vi "sc5511a_soft_front_panel.vi"() -> ()   [LabVIEW 2010]
panel:
  out "message":string="List/Sweep Mode Disabled"
  out "Selected Resource":string
  out "On":bool
  in  "stop":bool
  in  "Tab Control":T1(tab)
  in  "Spur Suppression":u8(ring) items=["Enabled", "Disabled"]
  in  "AutoLevel":u8(ring) items=["Enable", "Disable"]
  in  "Loop Gain":u8(ring) items=["Normal", "Low"]
  in  "Ref. Out Freq":u8(ring) items=["10 MHz", "100 MHz"]
  in  "Ref. Clock Source":u8(ring) items=["Internal 10 MHz", "Lock to External"]
  in  "RF1 Standby":bool
  in  "Lock Mode":u8(ring) items=["Harmonic Lock", "Frac-N Lock"]
  in  "ALC MODE":u8(ring) items=["Closed", "Opened"]
  in  "Power":sgl=30.0 min=-40 max=30 format="%.2f"
  in  "Interval (s)":u16=5
  in  "GetStatus":bool
  in  "Trigger":bool
  out "Device Status":T2={"Synth Mode"=1, "RF Out"=0, "Auto Level"=0, "ALC Mode"=1, "Standby"=1, "Rf RF Mode"=0, "List Mode State"=0, "RF2 Standby"=0, "Ref Lock Enable"=1, "Ext Ref Detected"=1, "Ref out mode"=1, "Main PLL"=1, "Crs PLL"=1, "Fine PLL"=1, "device accessed"=0, "Over Temp"=0, "MainLED"=FALSE, "CrsLED"=FALSE, "FineLED"=FALSE} {"Over Temp" items=["Normal", "Over Temp"]; "Ref out mode" items=["10 MHz", "100 MHz"]; "device accessed" items=["NO", "YES"]; "RF2 Standby" items=["Disabled", "Enabled"]; "Standby" items=["Disable", "Enabled"]; "Auto Level" items=["Enable", "Disable"]; "Ext Ref Detected" items=["Not Detected", "Detected"]; "Ref Lock Enable" items=["Disabled", "Enabled"]; "RF Out" items=["Disabled", "Enabled"]; "ALC Mode" items=["Closed", "Opened"]; "Rf RF Mode" items=["Single Tone", "List/Sweep"]; "Synth Mode" items=["Harmonic", "FracN"]; "List Mode State" items=["Not Triggered", "Triggered"]; "Main PLL" items=["NOT Locked", "Locked"]; "Crs PLL" items=["NOT Locked", "Locked"]; "Fine PLL" items=["NOT Locked", "Locked"]}
  in  "RF Frequency":dbl=2005000000.0 min=80000000.0 max=21000000000.0 step=1.0 format="%.9p"
  in  "RF Mode":u8(ring) items=["Single Tone", "List/Sweep"]
  in  "RF Enable":bool
  in  "RF2 Freq":sgl=6000.0 min=25 max=6000 step=25
  in  "RF2 Standby":bool
  in  "Set As Default":bool
  in  "Dwell Period (ms)":dbl=10.0 min=0.0 step=0.5 format="%.1f"
  in  "Sweep/List Cycles":u32
  in  "Sweep Freq Parameter":T3={"Start Frequency"=10040000000, "Stop Frequency"=10050000000, "Step Frequency"=100000} {"Step Frequency" max=6500000000 format="%.9p"; "Stop Frequency" max=21000000000 format="%.9p"; "Start Frequency" format="%.9p"}
  in  "List Mode Config":T4={"Sweep / List"=1, "Direction"=0, "Shape"=1, "Trigger Source"=1, "HW Trigger Mode"=0, "Return to Start"=0, "Trigger Out State"=1, "Trigger Out Behavior"=0} {"Trigger Out Behavior" items=["Trigger On Step", "Trigger On Cycle"]; "Trigger Out State" items=["Trigger Out Disable", "Trigger Out Enable"]; "Return to Start" items=["Stop at End", "Return to Start"]; "HW Trigger Mode" items=["Start/Stop", "Step"]; "Trigger Source" items=["Software", "Hardware"]; "Shape" items=["Sawtooth", "Triangle"]; "Direction" items=["Low to High", "High to Low"]; "Sweep / List" items=["List", "Sweep (start/stop/step)"]}
  in  "Load Config":bool
  in  "Save Buffer to EEPROM":bool
  in  "Read EEPROM to Buffer":bool
  in  "Download to Buffer":bool
  in  "Read From File":bool
  in  "Frequency List (2048 max)":u64[](array[numeric]) format="%.9p"
  out "message 2":string
  out "List Points":u32
  in  "SelfCal":bool
  out "Temperature":sgl=40.0 min=-30 max=120 format="%.1f"
  out "Device Info":T5={"Product SN"=268435879, "Hardware Rev"=2.0, "Firmware Rev"=2.0, "Manuf Date"={"Year"=14, "Month"=9, "Day"=10, "Hour"=10}} {"Firmware Rev" format="%.2g"; "Hardware Rev" format="%.2g"; "Product SN" format="%.0x"}
  out "error out":errorcluster
  # "MHz"
  # "Program will stop and the device will \nreinitialize after self calibration"
  # "DegC"
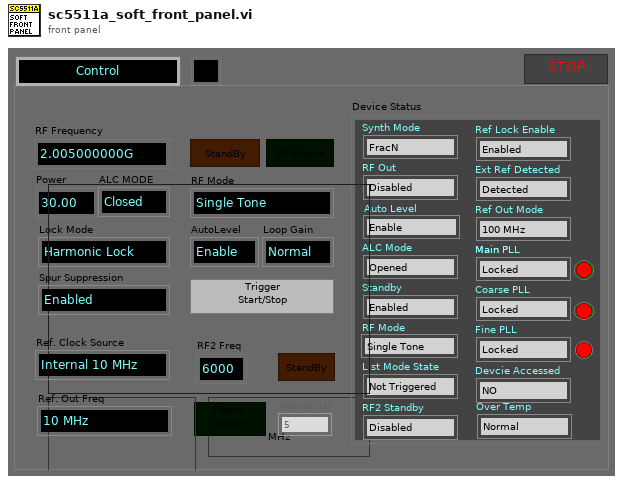
[diagram p1: front panel]
types:
  T1 = enum32{"Control", "Config Sweep/List", "List Entry", "Device Info"}
  T2 = cluster{"Synth Mode":u16, "RF Out":u16, "Auto Level":u16, "ALC Mode":u16, "Standby":u16, "Rf RF Mode":u16, "List Mode State":u16, "RF2 Standby":u16, "Ref Lock Enable":u16, "Ext Ref Detected":u16, "Ref out mode":u16, "Main PLL":u8, "Crs PLL":u8, "Fine PLL":u8, "device accessed":u16, "Over Temp":u16, "MainLED":bool, "CrsLED":bool, "FineLED":bool}
  T3 = cluster{"Start Frequency":u64, "Stop Frequency":u64, "Step Frequency":u64}
  T4 = cluster{"Sweep / List":u8, "Direction":u8, "Shape":u8, "Trigger Source":u8, "HW Trigger Mode":u8, "Return to Start":u8, "Trigger Out State":u8, "Trigger Out Behavior":u8}
  T5 = cluster{"Product SN":u32, "Hardware Rev":sgl, "Firmware Rev":sgl, "Manuf Date":cluster{"Year":u8, "Month":u8, "Day":u8, "Hour":u8}}
  T6 = cluster{"Product SN":u32, "Hardware Rev":sgl, "Firmware Rev":sgl, "Manuf Date":cluster{"Year":u32, "Month":u32, "Day":u32, "hour":u32}}
  T7 = enum32{"Control", "Config Sweep/List", "List Entry"}
  T8 = enum8{"Enabled", "Disabled", "Disabled and Grayed Out"}
  T9 = cluster{"Synth Mode":u16, "RF Out":u16, "Auto Power":u16, "ALC Mode":u16, "Standby":u16, "Rf RF Mode":u16, "List Mode State":u16, "RF2 Standby":u16, "Ref Lock Enable":u16, "Ext Ref Detected":u16, "Ref out mode":u16, "Main PLL":u8, "Crs PLL":u8, "Fine PLL":u8, "device accessed":u16, "Over Temp":u16, "MainLED":bool, "CrsLED":bool, "FineLED":bool}
  T10 = cluster{"Product SN":u32, "Hardware Rev":sgl, "Firmware Rev":sgl, "Manufacture Date":cluster{"Year":u8, "Month":u8, "Day":u8, "hour":u8}}
  T11 = cluster{"List Mode Config":cluster{"List/SSS":u8, "Direction":u8, "Shape":u8, "Trigger Source":u8, "HW Trigger Mode":u8, "Return to Start":u8, "Trigger Out State":u8, "Trigger Out Behavior":u8}, "Operate Status":cluster{"Lock Mode":u8, "Loop Gain":u8, "Device Accessed":u8, "RF2 Standby":u8, "RF1 Standby":u8, "AutoPwrLevel":u8, "AlcMode":u8, "RFOutState":u8, "Ref Lock Enable":u8, "ExtRefDetected":u8, "RefOutSelect":u8, "ListRuning":u8, "RF Mode":u8, "OverTempStatus":u8, "Harmonic_SS":u8}, "PLL Status":cluster{"Sum PLL":u8, "Crs PLL":u8, "Fine PLL":u8, "Crs Ref PLL":u8, "Crs assist PLL":u8, "Ref Clk PLL":u8, "Clk 10 PLL":u8, "Lo2 PLL":u8}}
  T12 = cluster{"RF1 Freq":u64, "Sweep Start Freq":u64, "Sweep Stop Freq":u64, "Sweep Step Freq":u64, "Sweep dwell time (.5ms)":u32, "Sweep Cycles":u32, "List Buffer Points":u32, "RF1 Level (dBm)":sgl, "RF2 freq":u16}
  T13 = cluster{"List/SSS":u8, "Direction":u8, "Shape":u8, "Trigger Source":u8, "HW Trigger Mode":u8, "Return to Start":u8, "Trigger Out State":u8, "Trigger Out Behavior":u8}
  T14 = cluster{"Sweep Start Freq":u64, "Sweep Stop Freq":u64, "Sweep Step Freq":u64}
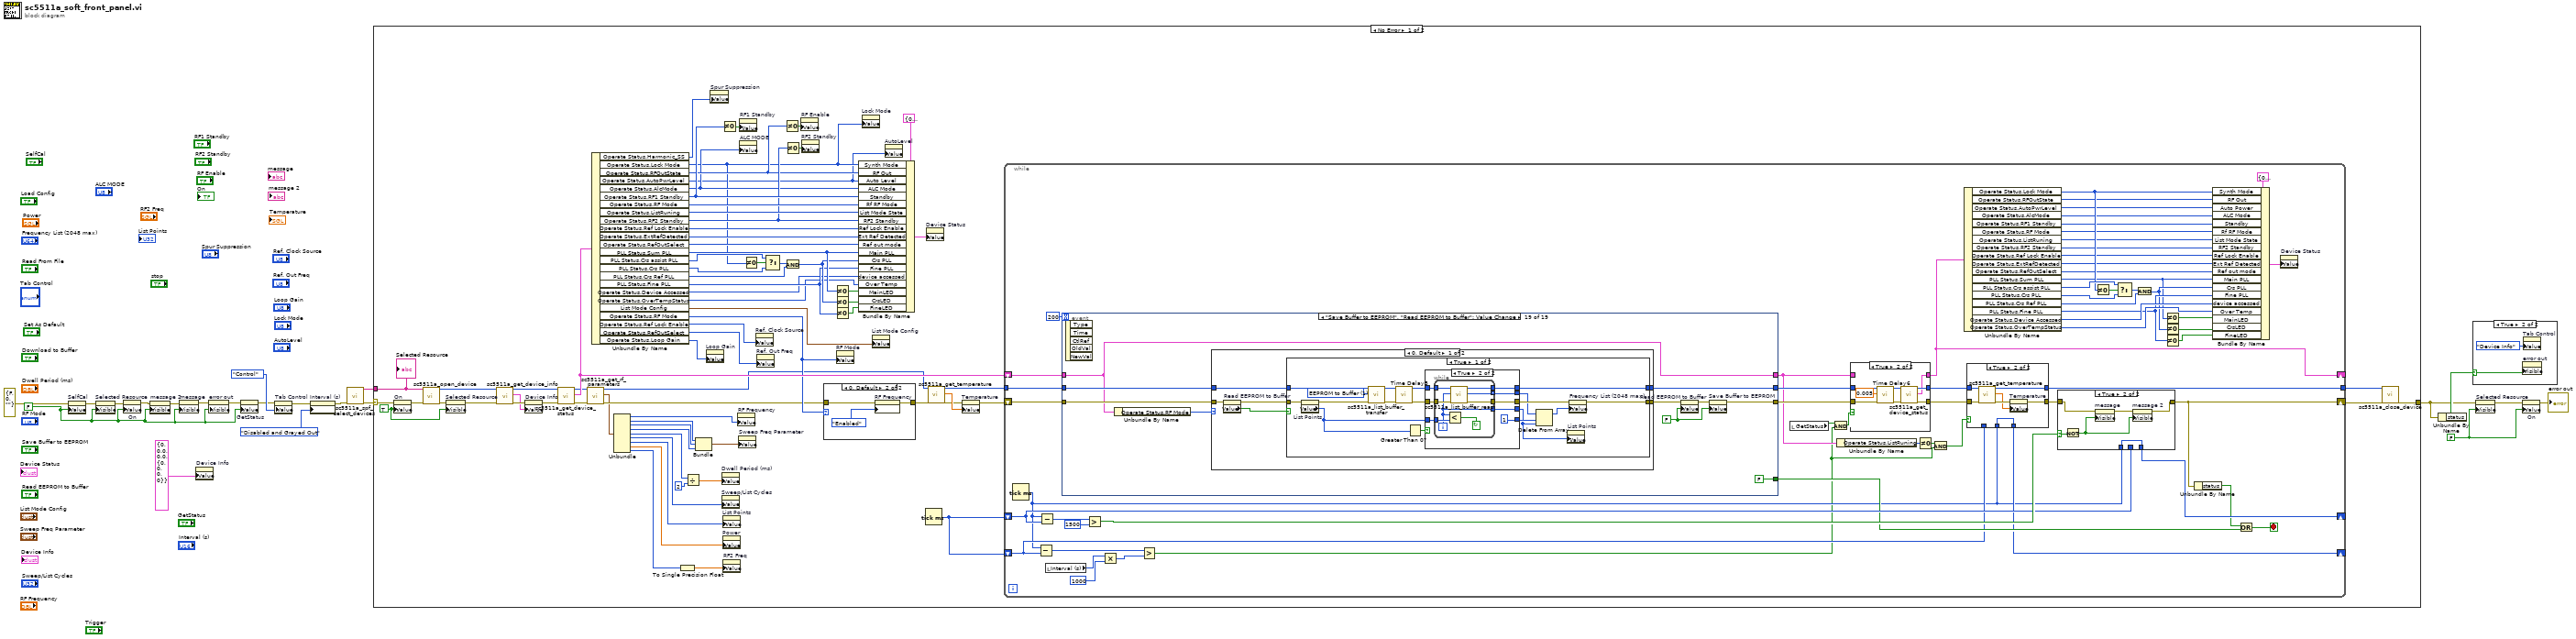
[diagram p0: block diagram]
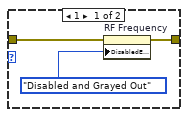
[diagram p3: hidden frame]
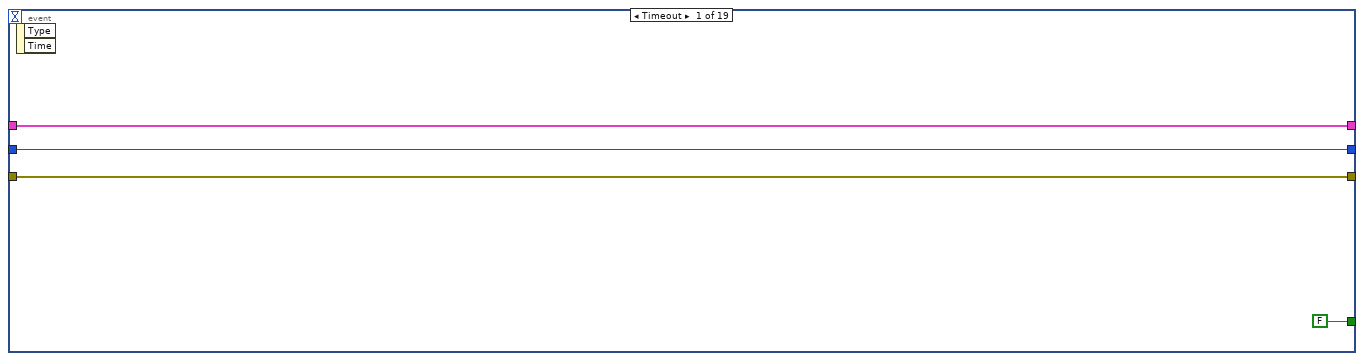
[diagram p7: hidden frame]
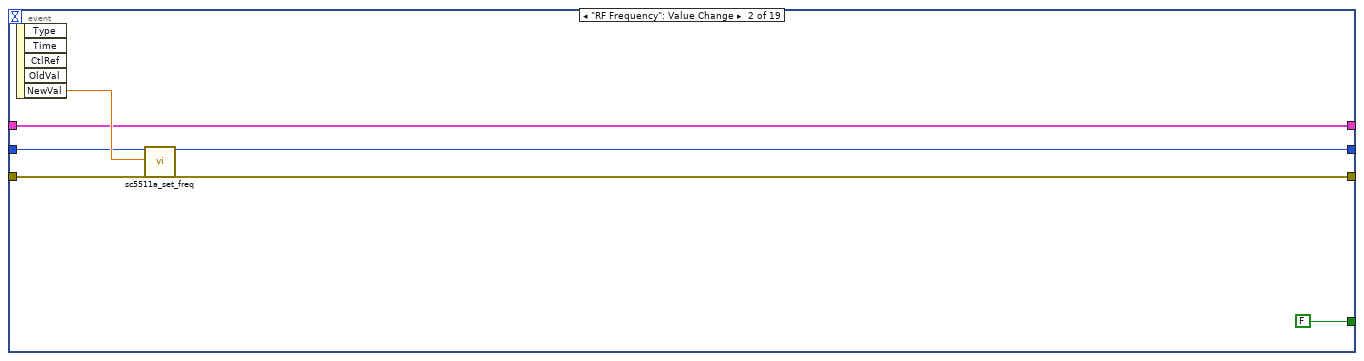
[diagram p8: hidden frame]
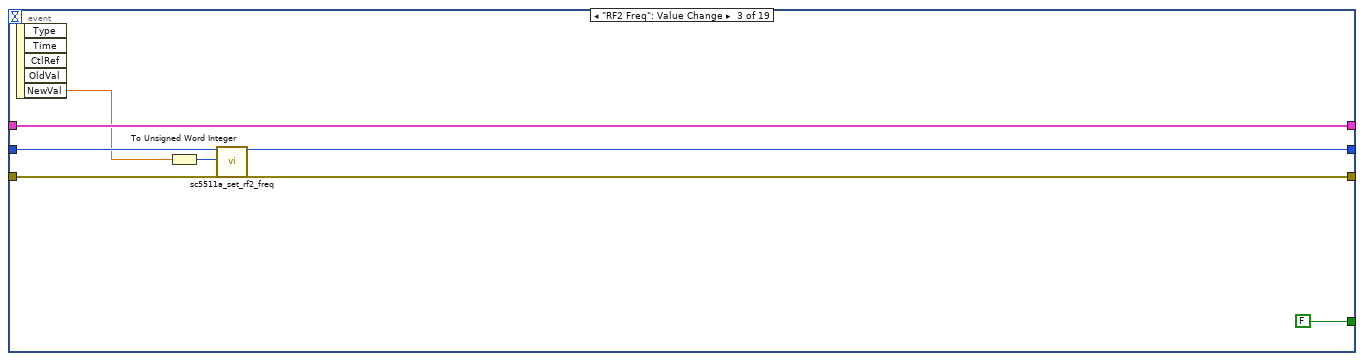
[diagram p9: hidden frame]
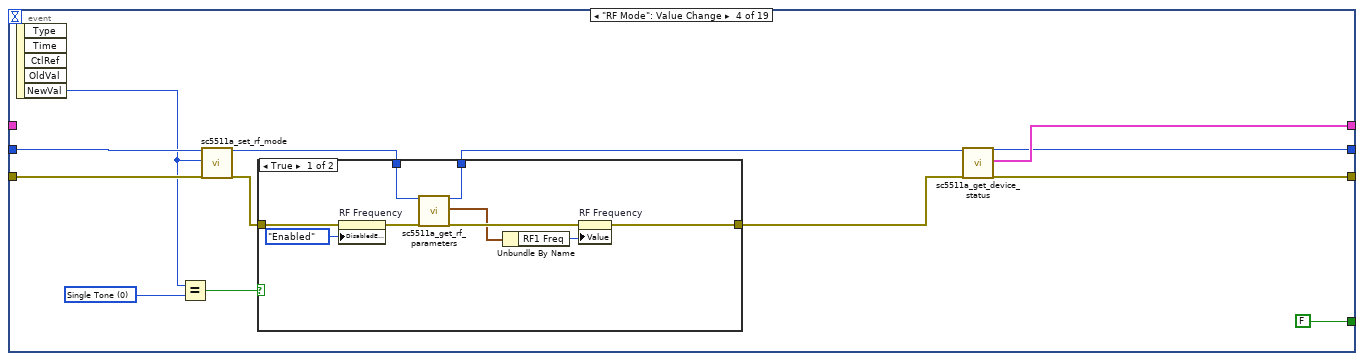
[diagram p10: hidden frame]
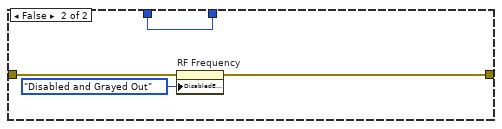
[diagram p11: hidden frame]
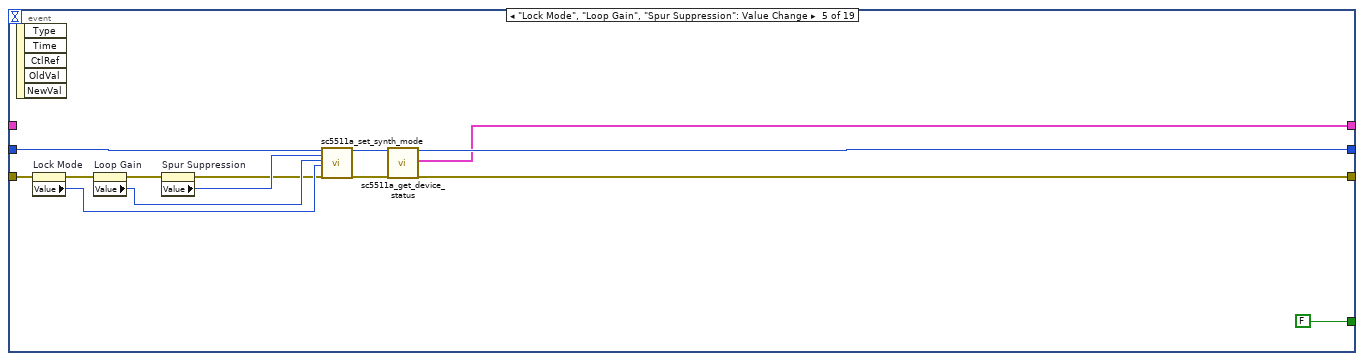
[diagram p12: hidden frame]
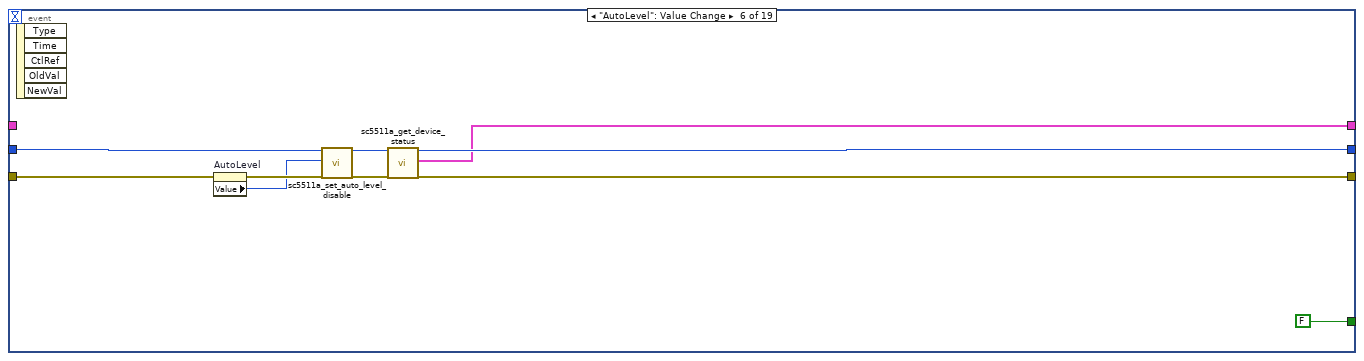
[diagram p13: hidden frame]
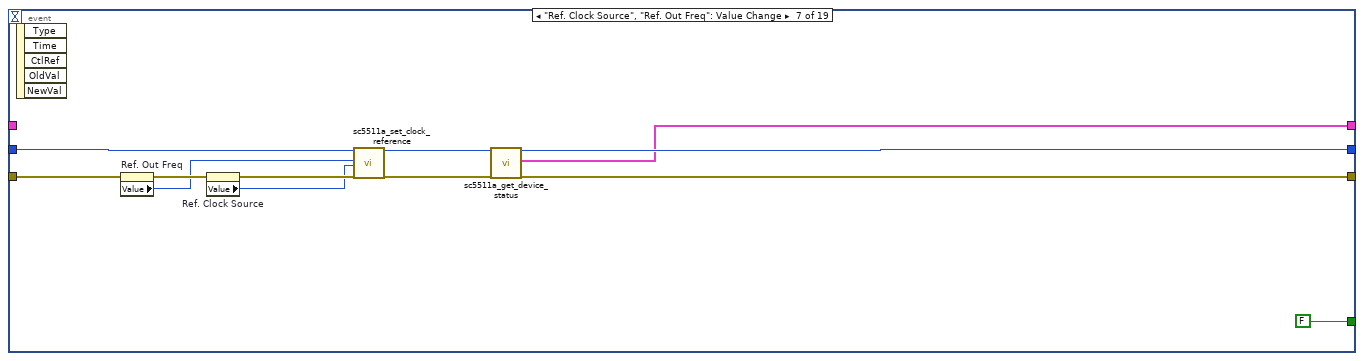
[diagram p14: hidden frame]
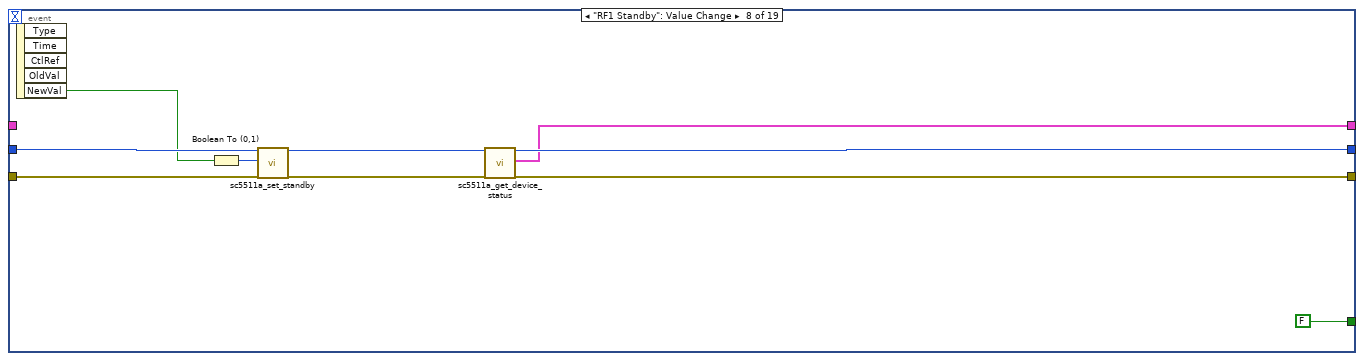
[diagram p15: hidden frame]
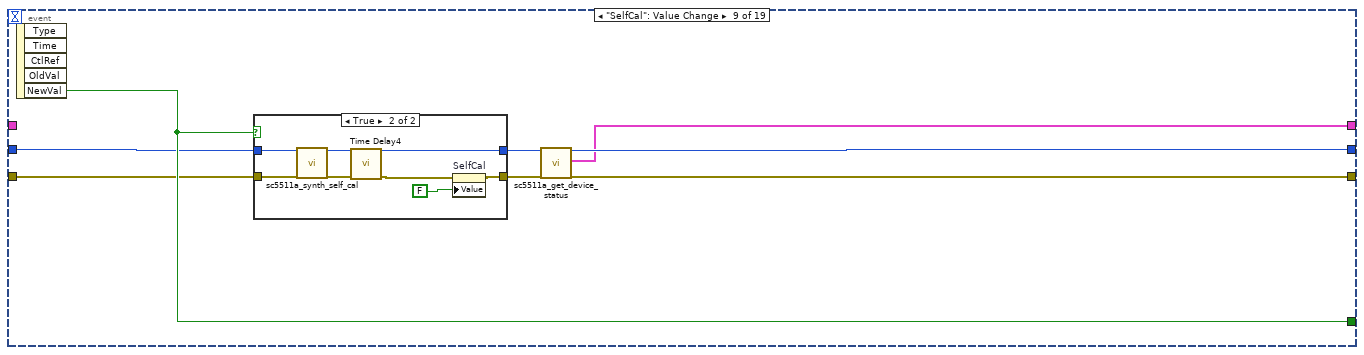
[diagram p16: hidden frame]
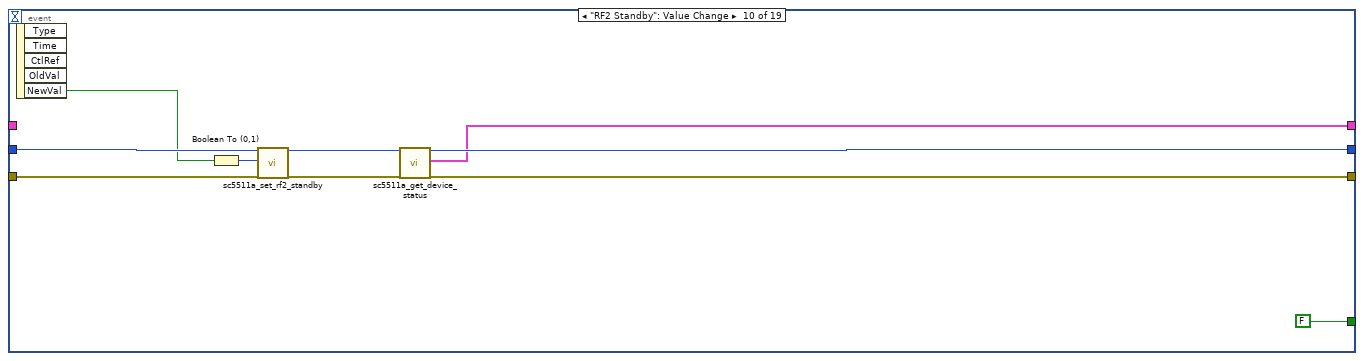
[diagram p18: hidden frame]
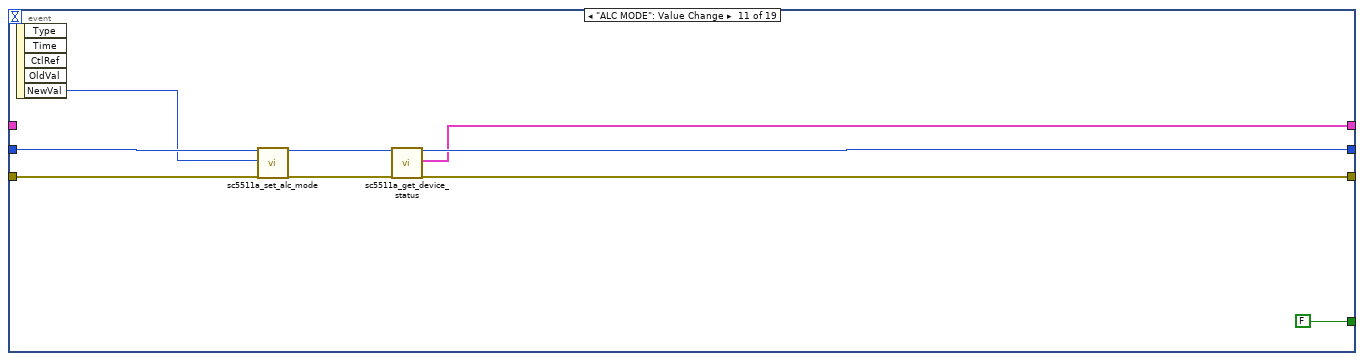
[diagram p19: hidden frame]
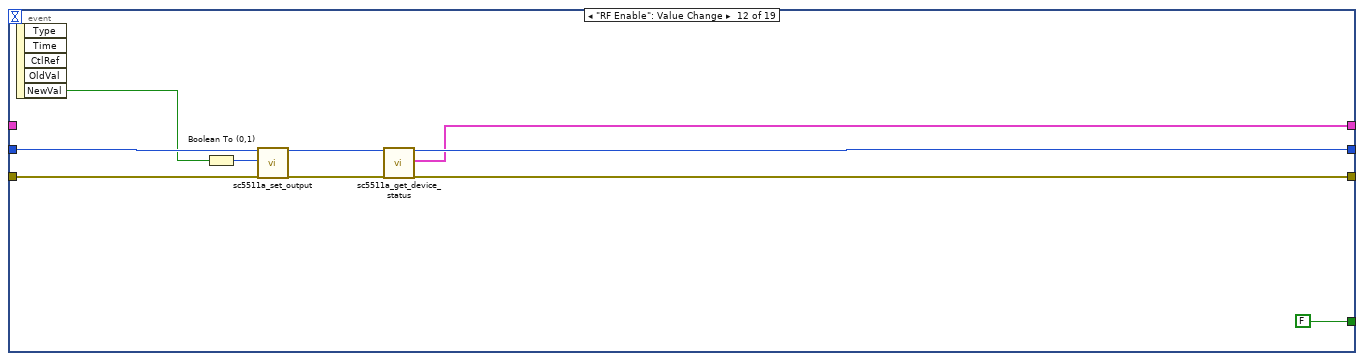
[diagram p20: hidden frame]
diagram:
  w4 = FALSE ("Visible")
  w2 = FALSE ("Visible")
  n1 = property on="SelfCal" class="Bool (strict)"(error in=errorcluster {"status"=FALSE, "code"=0, "source"=""} ("error in (no error)"), "Value"=w2) -> (error out=w3:errorcluster)  [unwired: 1 in, 1 out]
  n2 = property on="Selected Resource" class="Str"(error in=w3, "Visible"=w2) -> (error out=w7:errorcluster)  [unwired: 1 in, 1 out]
  n3 = property on="On" class="Bool (strict)"(error in=w7, "Value"=w2) -> (error out=w12:errorcluster)  [unwired: 1 in, 1 out]
  n4 = property on="message 2" class="Str"(error in=w12, "Visible"=w2) -> (error out=w21:errorcluster)  [unwired: 1 in, 1 out]
  n5 = property on="message" class="Str"(error in=w21, "Visible"=w2) -> (error out=w20:errorcluster)  [unwired: 1 in, 1 out]
  n6 = property on="Device Info" class="Clust (strict)"("Value"=T6 {"Product SN"=0, "Hardware Rev"=0.0, "Firmware Rev"=0.0, "Manuf Date"={"Year"=0, "Month"=0, "Day"=0, "hour"=0}} ("Device Info")) -> ()  [unwired: 2 in, 2 out]
  n7 = property on="error out" class="Clust (strict)"(error in=w20, "Visible"=w2) -> (error out=w19:errorcluster)  [unwired: 1 in, 1 out]
  n8 = property on="GetStatus" class="Bool (strict)"(error in=w19, "Value"=w2) -> (error out=w15:errorcluster)  [unwired: 1 in, 1 out]
  n9 = property on="Tab Control" class="TabCtl (strict)"(error in=w15, "Value"=T7."Control" ("Tab Control")) -> (error out=w16:errorcluster)  [unwired: 1 in, 1 out]
  n10 = property on="Interval (s)" class="DigNum (strict)"(error in=w16, "DisabledEnum"=T8."Disabled and Grayed Out" ("Disabled")) -> (error out=w9:errorcluster)  [unwired: 1 in, 1 out]
  n11 = call "sc5511a_spf_select_devices.vi"("error in (no error)"=w9) -> ("Selected Resource"=w8:string, "error out"=w10:errorcluster)  [unwired: 17 in]
  n12 = case shown="No Error" w10 {
    selector: w10 -> [w80 w556]
    tunnel: [w93 w556] -> w6
    tunnel: w8 -> [w79 _]
    frame No Error {
      w23 = TRUE ("Visible")
      n13 = property on="On" class="Bool (strict)"(error in=w80, "Value"=w23) -> (error out=w81:errorcluster)  [unwired: 1 in, 1 out]
      n14 = call "sc5511a_open_device.vi"("COM (String) eg COM1"=w79, "error in (no error)"=w81) -> ("deviceHandle"=w83:u32, "error out"=w25:errorcluster)  [unwired: 16 in]
      n15 = property on="Selected Resource" class="Str"(error in=w25, "Visible"=w23) -> (error out=w24:errorcluster)  [unwired: 1 in, 1 out]
      n16 = call "sc5511a_get_device_info.vi"("deviceHandle"=w83, "error in"=w24) -> ("deviceHandle"=w90:u32, "Device Info"=w75:T10, "error out"=w89:errorcluster)  [unwired: 15 in]
      n17 = property on="Device Info" class="Clust (strict)"(error in=w89, "Value"=w75) -> (error out=w88:errorcluster)  [unwired: 1 in, 1 out]
      n18 = call "sc5511a_get_device_status.vi"("deviceHandle"=w90, "error in"=w88) -> ("deviceHandle"=w76:u32, "Device Status"=w91:T11, "error out"=w78:errorcluster)  [unwired: 15 in]
      n19 = call "sc5511a_get_rf_parameters.vi"("deviceHandle"=w76, "error in"=w78) -> ("deviceHandle"=w36:u32, "RF Params"=w74:T12, "error out"=w77:errorcluster)  [unwired: 15 in]
      n20 = Unbundle By Name(w91) -> ("Operate Status.Harmonic_SS"=w22:u8, "Operate Status.Lock Mode"=w29:u8, "Operate Status.RFOutState"=w38:u8, "Operate Status.AutoPwrLevel"=w26:u8, "Operate Status.AlcMode"=w37:u8, "Operate Status.RF1 Standby"=w43:u8, "Operate Status.RF Mode"=w60:u8, "Operate Status.ListRuning"=w59:u8, "Operate Status.RF2 Standby"=w39:u8, "Operate Status.Ref Lock Enable"=w58:u8, "Operate Status.ExtRefDetected"=w57:u8, "Operate Status.RefOutSelect"=w56:u8, "PLL Status.Sum PLL"=w55:u8, "PLL Status.Crs assist PLL"=w51:u8, "PLL Status.Crs PLL"=w50:u8, "PLL Status.Crs Ref PLL"=w52:u8, "PLL Status.Fine PLL"=w48:u8, "Operate Status.Device Accessed"=w47:u8, "Operate Status.OverTempStatus"=w46:u8, "List Mode Config"=w92:T13, "Operate Status.RF Mode"=w82:u8, "Operate Status.Ref Lock Enable"=w45:u8, "Operate Status.RefOutSelect"=w44:u8, "Operate Status.Loop Gain"=w30:u8)
      n21 = Unbundle(w74) -> ("RF1 Freq"=w73:u64, "Sweep Start Freq"=w71:u64, "Sweep Stop Freq"=w70:u64, "Sweep Step Freq"=w69:u64, "Sweep dwell time (.5ms)"=w66:u32, "Sweep Cycles"=w68:u32, "List Buffer Points"=w64:u32, "RF1 Level (dBm)"=w63:sgl, "RF2 freq"=w61:u16)
      n22 = To Single Precision Float(number=w61) -> (single precision float=w62:sgl)
      n23 = Divide(x=w66, y=u32 2) -> (x/y=w67:dbl)
      n24 = Bundle("Sweep Start Freq"=w71, "Sweep Stop Freq"=w70, "Sweep Step Freq"=w69) -> (w72:T14)  [unwired: 1 in]
      n25 = property on="Loop Gain" class="Ring (strict)"("Value"=w30) -> ()  [unwired: 2 in, 2 out]
      n26 = property on="Spur Suppression" class="Ring (strict)"("Value"=w22) -> ()  [unwired: 2 in, 2 out]
      n27 = Not Equal To 0?(x=w43) -> (x != 0?=w42:bool)
      n28 = property on="Dwell Period (ms)" class="DigNum (strict)"("Value"=w67) -> ()  [unwired: 2 in, 2 out]
      n29 = property on="Sweep/List Cycles" class="DigNum (strict)"("Value"=w68) -> ()  [unwired: 2 in, 2 out]
      n30 = property on="Power" class="DigNum (strict)"("Value"=w63) -> ()  [unwired: 2 in, 2 out]
      n31 = property on="List Points" class="DigNum (strict)"("Value"=w64) -> ()  [unwired: 2 in, 2 out]
      n32 = property on="RF2 Freq" class="DigNum (strict)"("Value"=w62) -> ()  [unwired: 2 in, 2 out]
      n33 = property on="RF Frequency" class="DigNum (strict)"("Value"=w73) -> ()  [unwired: 2 in, 2 out]
      n34 = property on="Sweep Freq Parameter" class="Clust (strict)"("Value"=w72) -> ()  [unwired: 2 in, 2 out]
      n35 = property on="RF1 Standby" class="Bool (strict)"("Value"=w42) -> ()  [unwired: 2 in, 2 out]
      n36 = property on="ALC MODE" class="Ring (strict)"("Value"=w37) -> ()  [unwired: 2 in, 2 out]
      n37 = Not Equal To 0?(x=w29) -> (x != 0?=w54:bool)
      n38 = property on="Ref. Clock Source" class="Ring (strict)"("Value"=w45) -> ()  [unwired: 2 in, 2 out]
      n39 = property on="Ref. Out Freq" class="Ring (strict)"("Value"=w44) -> ()  [unwired: 2 in, 2 out]
      n40 = Select(t=w51, s=w54, f=w50) -> (s? t:f=w53:u8)
      n41 = Not Equal To 0?(x=w38) -> (x != 0?=w41:bool)
      n42 = Not Equal To 0?(x=w39) -> (x != 0?=w40:bool)
      n43 = And(x=w53, y=w52) -> (x .and. y?=w49:u8)
      n44 = property on="RF Enable" class="Bool (strict)"("Value"=w41) -> ()  [unwired: 2 in, 2 out]
      n45 = property on="RF2 Standby" class="Bool (strict)"("Value"=w40) -> ()  [unwired: 2 in, 2 out]
      n46 = case shown="0, Default" w82 {
        tunnel: w77 -> [w97 w100]
        tunnel: [w96 w99] -> w34
        frame 1 {
          n47 = property on="RF Frequency" class="DigNum (strict)"(error in=w97, "DisabledEnum"=T8."Disabled and Grayed Out" ("Disabled")) -> (error out=w96:errorcluster)  [unwired: 1 in, 1 out]
        }
        frame 0, Default {
          n48 = property on="RF Frequency" class="DigNum (strict)"(error in=w100, "DisabledEnum"=T8."Enabled" ("Disabled")) -> (error out=w99:errorcluster)  [unwired: 1 in, 1 out]
        }
      }
      n49 = Not Equal To 0?(x=w55) -> (x != 0?=w86:bool)
      n50 = Not Equal To 0?(x=w49) -> (x != 0?=w85:bool)
      n51 = Not Equal To 0?(x=w48) -> (x != 0?=w84:bool)
      n52 = property on="RF Mode" class="Ring (strict)"("Value"=w82) -> ()  [unwired: 2 in, 2 out]
      n53 = Bundle By Name(cluster=T2 {"Synth Mode"=0, "RF Out"=1, "Auto Level"=1, "ALC Mode"=0, "Standby"=0, "Rf RF Mode"=0, "List Mode State"=0, "RF2 Standby"=1, "Ref Lock Enable"=0, "Ext Ref Detected"=0, "Ref out mode"=0, "Main PLL"=1, "Crs PLL"=1, "Fine PLL"=1, "device accessed"=1, "Over Temp"=0, "MainLED"=TRUE, "CrsLED"=TRUE, "FineLED"=TRUE} ("Device Status"), "Synth Mode"=w29, "RF Out"=w38, "Auto Level"=w26, "ALC Mode"=w37, "Standby"=w43, "Rf RF Mode"=w60, "List Mode State"=w59, "RF2 Standby"=w39, "Ref Lock Enable"=w58, "Ext Ref Detected"=w57, "Ref out mode"=w56, "Main PLL"=w55, "Crs PLL"=w49, "Fine PLL"=w48, "device accessed"=w47, "Over Temp"=w46, "MainLED"=w86, "CrsLED"=w85, "FineLED"=w84) -> (w28:T2)
      n54 = property on="Lock Mode" class="Ring (strict)"("Value"=w29) -> ()  [unwired: 2 in, 2 out]
      n55 = property on="List Mode Config" class="Clust (strict)"("Value"=w92) -> ()  [unwired: 2 in, 2 out]
      n56 = property on="AutoLevel" class="Ring (strict)"("Value"=w26) -> ()  [unwired: 2 in, 2 out]
      n57 = Tick Count (ms)() -> (millisecond timer value=w87:u32)
      n58 = property on="Device Status" class="Clust (strict)"("Value"=w28) -> ()  [unwired: 2 in, 2 out]
      n59 = call "sc5511a_get_temperature.vi"("deviceHandle"=w36, "error in"=w34) -> ("deviceHandle"=w35:u32, "temperature"=w33:sgl, "error out"=w31:errorcluster)  [unwired: 15 in]
      n60 = property on="Temperature" class="DigNum (strict)"(error in=w31, "Value"=w33) -> (error out=w32:errorcluster)  [unwired: 1 in, 1 out]
      n61 = while {
        shift-right: [w143] -> w95
        shift-left: w32 -> [w161]
        tunnel: w35 -> [w160]
        tunnel: [w110] -> w94
        shift-right: [w118] -> _
        shift-left: w91 -> [w157]
        shift-right: [w147] -> _
        shift-left: w87 -> [w146]
        shift-right: [w113] -> _
        shift-left: w87 -> [w114]
        stop <- w142 stop-if-true
        n62 = Tick Count (ms)() -> (millisecond timer value=w112:u32)
        n63 = Subtract(x=w112, y=w114) -> (x-y=w151:u32)
        n64 = Subtract(x=w112, y=w146) -> (x-y=w156:u32)
        n65 = local read "Interval (s)"() -> (w152:u16)
        n66 = event shown="[18] \"Save Buffer to EEPROM\", \"Read EEPROM to Buffer\": Value Change" {
          selector: _ -> [_ _ _ _ _ _ _ _ _ _ _ _ _ _ _ _ _ _ _]
          dyn-events: _ -> [_ _ _ _ _ _ _ _ _ _ _ _ _ _ _ _ _ _ _]
          timeout: 200 -> [_ _ _ _ _ _ _ _ _ _ _ _ _ _ _ _ _ _ _]
          tunnel: w160 -> [w192 w199 w208 w219 w247 w257 w269 w278 w284 w305 w314 w324 w330 w335 w356 w367 w439 w454 w501]
          tunnel: w161 -> [w193 w198 w207 w220 w241 w249 w268 w279 w283 w306 w315 w325 w331 w340 w353 w368 w438 w455 w502]
          tunnel: [w192 w196 w205 w211 w244 w254 w260 w273 w287 w301 w310 w319 w329 w336 w356 w360 w415 w453 w496] -> w159
          tunnel: [w193 w197 w206 w212 w246 w256 w263 w274 w288 w302 w312 w321 w328 w337 w354 w362 w413 w452 w497] -> w158
          tunnel: w157 -> [w191 w195 w204 _ _ _ _ _ _ _ _ _ w333 _ w357 w363 w411 w447 w494]
          tunnel: [w191 w195 w204 w214 w242 w252 w259 w271 w286 w298 w308 w317 w333 w334 w357 w358 w411 w447 w494] -> w107
          tunnel: [FALSE ("NewVal") FALSE FALSE FALSE FALSE FALSE FALSE FALSE w285 FALSE FALSE FALSE FALSE FALSE TRUE ("NewVal") FALSE ("NewVal") FALSE ("NewVal") FALSE ("NewVal") FALSE ("NewVal")] -> w145
          event Timeout {
            n67 = event-data() -> ()  [unwired: 1 in, 2 out]
          }
          event "RF Frequency": Value Change {
            n68 = event-data() -> ("NewVal"=w200:dbl)  [unwired: 1 in, 4 out]
            n69 = call "sc5511a_set_freq.vi"("deviceHandle"=w199, "RF1 frequency"=w200, "error in"=w198) -> ("deviceHandle"=w196:u32, "error out"=w197:errorcluster)  [unwired: 15 in]
          }
          event "RF2 Freq": Value Change {
            n70 = event-data() -> ("NewVal"=w201:sgl)  [unwired: 1 in, 4 out]
            n71 = To Unsigned Word Integer(number=w201) -> (unsigned 16bit integer=w202:u16)
            n72 = call "sc5511a_set_rf2_freq.vi"("deviceHandle"=w208, "RF1 frequency (MHz)"=w202, "error in"=w207) -> ("deviceHandle"=w205:u32, "error out"=w206:errorcluster)  [unwired: 15 in]
          }
          event "RF Mode": Value Change {
            w217 = u8 0 items=["Single Tone", "List/Sweep"] ("RF Mode")
            n73 = event-data() -> ("NewVal"=w216:u8)  [unwired: 1 in, 4 out]
            n74 = Equal?(x=w216, y=w217) -> (x = y?=w215:bool)
            n75 = call "sc5511a_set_rf_mode.vi"("deviceHandle"=w219, "RF Mode"=w216, "error in"=w220) -> ("deviceHandle"=w210:u32, "error out"=w218:errorcluster)  [unwired: 15 in]
            n76 = case shown="True" w215 {
              tunnel: w218 -> [w230 w234]
              tunnel: [w226 w233] -> w213
              tunnel: [w223 w231] -> w209
              tunnel: w210 -> [w222 w231]
              frame True {
                n77 = property on="RF Frequency" class="DigNum (strict)"(error in=w230, "DisabledEnum"=T8."Enabled" ("Disabled")) -> (error out=w228:errorcluster)  [unwired: 1 in, 1 out]
                n78 = call "sc5511a_get_rf_parameters.vi"("deviceHandle"=w222, "error in"=w228) -> ("deviceHandle"=w223:u32, "RF Params"=w225:T12, "error out"=w227:errorcluster)  [unwired: 15 in]
                n79 = Unbundle By Name(w225) -> ("RF1 Freq"=w224:u64)
                n80 = property on="RF Frequency" class="DigNum (strict)"(error in=w227, "Value"=w224) -> (error out=w226:errorcluster)  [unwired: 1 in, 1 out]
              }
              frame False {
                n81 = property on="RF Frequency" class="DigNum (strict)"(error in=w234, "DisabledEnum"=T8."Disabled and Grayed Out" ("Disabled")) -> (error out=w233:errorcluster)  [unwired: 1 in, 1 out]
              }
            }
            n82 = call "sc5511a_get_device_status.vi"("deviceHandle"=w209, "error in"=w213) -> ("deviceHandle"=w211:u32, "Device Status"=w214:T11, "error out"=w212:errorcluster)  [unwired: 15 in]
          }
          event "Lock Mode", "Loop Gain", "Spur Suppression": Value Change {
            n83 = event-data() -> ()  [unwired: 1 in, 5 out]
            n84 = property on="Lock Mode" class="Ring (strict)"(error in=w241) -> (error out=w240:errorcluster, "Value"=w238:u8)  [unwired: 1 in, 1 out]
            n85 = property on="Loop Gain" class="Ring (strict)"(error in=w240) -> (error out=w235:errorcluster, "Value"=w239:u8)  [unwired: 1 in, 1 out]
            n86 = property on="Spur Suppression" class="Ring (strict)"(error in=w235) -> (error out=w236:errorcluster, "Value"=w237:u8)  [unwired: 1 in, 1 out]
            n87 = call "sc5511a_set_synth_mode.vi"("deviceHandle"=w247, "Harmonic Spur Suppression"=w237, "loop gain"=w239, "lock mode"=w238, "error in"=w236) -> ("deviceHandle"=w243:u32, "error out"=w245:errorcluster)  [unwired: 13 in]
            n88 = call "sc5511a_get_device_status.vi"("deviceHandle"=w243, "error in"=w245) -> ("deviceHandle"=w244:u32, "Device Status"=w242:T11, "error out"=w246:errorcluster)  [unwired: 15 in]
          }
          event "AutoLevel": Value Change {
            n89 = event-data() -> ()  [unwired: 1 in, 5 out]
            n90 = property on="AutoLevel" class="Ring (strict)"(error in=w249) -> (error out=w251:errorcluster, "Value"=w250:u8)  [unwired: 1 in, 1 out]
            n91 = call "sc5511a_set_auto_level_disable.vi"("deviceHandle"=w257, "auto leveling"=w250, "error in"=w251) -> ("deviceHandle"=w253:u32, "error out"=w255:errorcluster)  [unwired: 15 in]
            n92 = call "sc5511a_get_device_status.vi"("deviceHandle"=w253, "error in"=w255) -> ("deviceHandle"=w254:u32, "Device Status"=w252:T11, "error out"=w256:errorcluster)  [unwired: 15 in]
          }
          event "Ref. Clock Source", "Ref. Out Freq": Value Change {
            n93 = event-data() -> ()  [unwired: 1 in, 5 out]
            n94 = property on="Ref. Out Freq" class="Ring (strict)"(error in=w268) -> (error out=w267:errorcluster, "Value"=w264:u8)  [unwired: 1 in, 1 out]
            n95 = property on="Ref. Clock Source" class="Ring (strict)"(error in=w267) -> (error out=w266:errorcluster, "Value"=w265:u8)  [unwired: 1 in, 1 out]
            n96 = call "sc5511a_set_clock_reference.vi"("deviceHandle"=w269, "Ref Output"=w264, "Lock external"=w265, "error in"=w266) -> ("deviceHandle"=w261:u32, "error out"=w262:errorcluster)  [unwired: 14 in]
            n97 = call "sc5511a_get_device_status.vi"("deviceHandle"=w261, "error in"=w262) -> ("deviceHandle"=w260:u32, "Device Status"=w259:T11, "error out"=w263:errorcluster)  [unwired: 15 in]
          }
          event "RF1 Standby": Value Change {
            n98 = event-data() -> ("NewVal"=w277:bool)  [unwired: 1 in, 4 out]
            n99 = Boolean To (0,1)(Boolean=w277) -> (0, 1=w276:i16)
            n100 = call "sc5511a_set_standby.vi"("deviceHandle"=w278, "Standby"=w276, "error in"=w279) -> ("deviceHandle"=w272:u32, "error out"=w275:errorcluster)  [unwired: 15 in]
            n101 = call "sc5511a_get_device_status.vi"("deviceHandle"=w272, "error in"=w275) -> ("deviceHandle"=w273:u32, "Device Status"=w271:T11, "error out"=w274:errorcluster)  [unwired: 15 in]
          }
          event "SelfCal": Value Change {
            n102 = event-data() -> ("NewVal"=w285:bool)  [unwired: 1 in, 4 out]
            n103 = case shown="True" w285 {
              tunnel: w284 -> [w290 w296]
              tunnel: w283 -> [w289 w297]
              tunnel: [w290 w294] -> w282
              tunnel: [w289 w293] -> w281
              frame False {
              }
              frame True {
                n104 = call "sc5511a_synth_self_cal.vi"("deviceHandle"=w296, "error in"=w297) -> ("deviceHandle"=w294:u32, "error out"=w295:errorcluster)  [unwired: 16 in]
                n105 = call "Time Delay4"("error in (no error)"=w295) -> ("error out"=w292:errorcluster)  [unwired: 10 in]
                n106 = property on="SelfCal" class="Bool (strict)"(error in=w292, "Value"=FALSE ("SelfCal")) -> (error out=w293:errorcluster)  [unwired: 1 in, 1 out]
              }
            }
            n107 = call "sc5511a_get_device_status.vi"("deviceHandle"=w282, "error in"=w281) -> ("deviceHandle"=w287:u32, "Device Status"=w286:T11, "error out"=w288:errorcluster)  [unwired: 15 in]
          }
          event "RF2 Standby": Value Change {
            n108 = event-data() -> ("NewVal"=w304:bool)  [unwired: 1 in, 4 out]
            n109 = Boolean To (0,1)(Boolean=w304) -> (0, 1=w303:i16)
            n110 = call "sc5511a_set_rf2_standby.vi"("deviceHandle"=w305, "Standby"=w303, "error in"=w306) -> ("deviceHandle"=w300:u32, "error out"=w299:errorcluster)  [unwired: 15 in]
            n111 = call "sc5511a_get_device_status.vi"("deviceHandle"=w300, "error in"=w299) -> ("deviceHandle"=w301:u32, "Device Status"=w298:T11, "error out"=w302:errorcluster)  [unwired: 15 in]
          }
          event "ALC MODE": Value Change {
            n112 = event-data() -> ("NewVal"=w313:u8)  [unwired: 1 in, 4 out]
            n113 = call "sc5511a_set_alc_mode.vi"("deviceHandle"=w314, "alc mode"=w313, "error in"=w315) -> ("deviceHandle"=w309:u32, "error out"=w311:errorcluster)  [unwired: 15 in]
            n114 = call "sc5511a_get_device_status.vi"("deviceHandle"=w309, "error in"=w311) -> ("deviceHandle"=w310:u32, "Device Status"=w308:T11, "error out"=w312:errorcluster)  [unwired: 15 in]
          }
          event "RF Enable": Value Change {
            n115 = event-data() -> ("NewVal"=w322:bool)  [unwired: 1 in, 4 out]
            n116 = Boolean To (0,1)(Boolean=w322) -> (0, 1=w323:i16)
            n117 = call "sc5511a_set_output.vi"("deviceHandle"=w324, "RF Output"=w323, "error in"=w325) -> ("deviceHandle"=w318:u32, "error out"=w320:errorcluster)  [unwired: 15 in]
            n118 = call "sc5511a_get_device_status.vi"("deviceHandle"=w318, "error in"=w320) -> ("deviceHandle"=w319:u32, "Device Status"=w317:T11, "error out"=w321:errorcluster)  [unwired: 15 in]
          }
          event "Power": Value Change {
            n119 = event-data() -> ("NewVal"=w327:sgl)  [unwired: 1 in, 4 out]
            n120 = call "sc5511a_set_level.vi"("deviceHandle"=w330, "level (dBm)"=w327, "error in"=w331) -> ("deviceHandle"=w329:u32, "error out"=w328:errorcluster)  [unwired: 15 in]
          }
          event "GetStatus": Value Change {
            n121 = event-data() -> ("NewVal"=w339:bool)  [unwired: 1 in, 4 out]
            n122 = case shown="True" w339 {
              selector: w339 -> [w345 w348]
              tunnel: w340 -> [w347 w351]
              tunnel: [w342 w350] -> w338
              tunnel: [w345 w348] -> _
              frame True {
                n123 = property on="RF Frequency" class="DigNum (strict)"(error in=w347, "DisabledEnum"=T8."Enabled" ("Disabled")) -> (error out=w343:errorcluster)  [unwired: 1 in, 1 out]
                n124 = property on="Interval (s)" class="DigNum (strict)"(error in=w343, "DisabledEnum"=T8."Enabled" ("Disabled")) -> (error out=w342:errorcluster)  [unwired: 1 in, 1 out]
              }
              frame False {
                n125 = property on="Interval (s)" class="DigNum (strict)"(error in=w351, "DisabledEnum"=T8."Disabled and Grayed Out" ("Disabled")) -> (error out=w350:errorcluster)  [unwired: 1 in, 1 out]
              }
            }
            n126 = call "sc5511a_get_device_status.vi"("deviceHandle"=w335, "error in"=w338) -> ("deviceHandle"=w336:u32, "Device Status"=w334:T11, "error out"=w337:errorcluster)  [unwired: 15 in]
          }
          event "stop": Value Change {
            n127 = event-data() -> ()  [unwired: 1 in, 5 out]
            n128 = property on="stop" class="Bool (strict)"(error in=w353, "Value"=FALSE ("stop")) -> (error out=w354:errorcluster)  [unwired: 1 in, 1 out]
          }
          event "Trigger": Value Change {
            (unwired) u16 0 ("ListMode State")
            n129 = event-data() -> ()  [unwired: 1 in, 5 out]
            n130 = Unbundle By Name(w363) -> ("Operate Status.RF Mode"=w371:u8, "Operate Status.ListRuning"=w370:u8, "List Mode Config.Trigger Source"=w369:u8)
            n131 = case shown="0, Default" w371 {
              tunnel: w370 -> [_ w383]
              tunnel: w369 -> [_ w382]
              tunnel: w368 -> [w374 w381]
              tunnel: [w373 w380] -> w365
              tunnel: w367 -> [w377 w379]
              tunnel: [w377 w378] -> w359
              frame 0, Default {
                n132 = property on="message" class="Str"(error in=w374, "Visible"=TRUE, "Value"="List/Sweep Mode Disabled" ("hwtrigSel'd")) -> (error out=w373:errorcluster)  [unwired: 1 in, 1 out]
              }
              frame 1 {
                n133 = case shown="1" w383 {
                  tunnel: w382 -> [w388 _]
                  tunnel: w381 -> [w387 w400]
                  tunnel: [w386 w399] -> w380
                  tunnel: w379 -> [w385 w401]
                  tunnel: [w384 w398] -> w378
                  frame 0, Default {
                    n134 = case shown="0, Default" w388 {
                      tunnel: [w391 w396] -> w386
                      tunnel: w387 -> [w392 w397]
                      tunnel: w385 -> [w390 w393]
                      tunnel: [w389 w393] -> w384
                      frame 0, Default {
                        n135 = call "sc5511a_list_soft_trigger.vi"("deviceHandle"=w390, "error in"=w392) -> ("deviceHandle"=w389:u32, "error out"=w391:errorcluster)  [unwired: 16 in]
                      }
                      frame 1 {
                        n136 = property on="message" class="Str"(error in=w397, "Visible"=TRUE, "Value"="Requires Hardware Tigger " ("hwtrigSel'd")) -> (error out=w396:errorcluster)  [unwired: 1 in, 1 out]
                      }
                    }
                  }
                  frame 1 {
                    n137 = call "sc5511a_list_soft_trigger.vi"("deviceHandle"=w401, "error in"=w400) -> ("deviceHandle"=w398:u32, "error out"=w399:errorcluster)  [unwired: 16 in]
                  }
                }
              }
            }
            n138 = call "Time Delay"("error in (no error)"=w365) -> ("error out"=w364:errorcluster)  [unwired: 10 in]
            n139 = property on="Trigger" class="Bool (strict)"(error in=w364, "Value"=FALSE ("Soft Tigger")) -> (error out=w361:errorcluster)  [unwired: 1 in, 1 out]
            n140 = call "sc5511a_get_device_status.vi"("deviceHandle"=w359, "error in"=w361) -> ("deviceHandle"=w360:u32, "Device Status"=w358:T11, "error out"=w362:errorcluster)  [unwired: 15 in]
          }
          event "Load Config", "Set As Default": Value Change {
            (unwired) u16 0 ("Direction")
            w412 = FALSE ("Soft Tigger")
            n141 = event-data() -> ()  [unwired: 1 in, 5 out]
            n142 = property on="List Mode Config" class="Clust (strict)"(error in=w438) -> (error out=w437:errorcluster, "Value"=w436:T4)  [unwired: 1 in, 1 out]
            n143 = call "sc5511a_list_mode_config.vi"("deviceHandle"=w439, "List Mode Config"=w436, "error in"=w437) -> ("deviceHandle"=w432:u32, "error out"=w435:errorcluster)  [unwired: 15 in]
            n144 = property on="Sweep Freq Parameter" class="Clust (strict)"(error in=w435) -> (error out=w429:errorcluster, "Value"=w434:T3)  [unwired: 1 in, 1 out]
            n145 = Unbundle(w434) -> ("Start Frequency"=w433:u64, "Stop Frequency"=w426:u64, "Step Frequency"=w425:u64)
            n146 = call "sc5511a_list_start_freq.vi"("deviceHandle"=w432, "List Start frequency"=w433, "error in"=w429) -> ("deviceHandle"=w431:u32, "error out"=w428:errorcluster)  [unwired: 15 in]
            n147 = call "sc5511a_list_stop_freq.vi"("deviceHandle"=w431, "RF frequency"=w426, "error in"=w428) -> ("deviceHandle"=w430:u32, "error out"=w427:errorcluster)  [unwired: 15 in]
            n148 = call "sc5511a_list_step_freq.vi"("deviceHandle"=w430, "List Step Frequency"=w425, "error in"=w427) -> ("deviceHandle"=w419:u32, "error out"=w424:errorcluster)  [unwired: 15 in]
            n149 = property on="Sweep/List Cycles" class="DigNum (strict)"(error in=w424) -> (error out=w422:errorcluster, "Value"=w423:u32)  [unwired: 1 in, 1 out]
            n150 = call "sc5511a_list_cycle_count.vi"("deviceHandle"=w419, "List Cycles"=w423, "error in"=w422) -> ("deviceHandle"=w418:u32, "error out"=w421:errorcluster)  [unwired: 15 in]
            n151 = property on="Dwell Period (ms)" class="DigNum (strict)"(error in=w421) -> (error out=w420:errorcluster, "Value"=w417:dbl)  [unwired: 1 in, 1 out]
            n152 = Multiply(x=w417, y=2.0) -> (x*y=w406:dbl)
            n153 = To Unsigned Long Integer(number=w406) -> (unsigned 32bit integer=w405:u32)
            n154 = call "sc5511a_list_dwell_time.vi"("deviceHandle"=w418, "List Dwell Time"=w405, "error in"=w420) -> ("deviceHandle"=w402:u32, "error out"=w403:errorcluster)  [unwired: 15 in]
            n155 = property on="Set As Default" class="Bool (strict)"(error in=w403) -> (error out=w416:errorcluster, "Value"=w414:bool)  [unwired: 1 in, 1 out]
            n156 = case shown="True" w414 {
              tunnel: w416 -> [w441 w445]
              tunnel: [w441 w444] -> w408
              tunnel: w402 -> [w440 w443]
              tunnel: [w440 w442] -> w415
              frame False {
              }
              frame True {
                n157 = call "sc5511a_store_default_state.vi"("deviceHandle"=w443, "error in"=w445) -> ("deviceHandle"=w442:u32, "error out"=w444:errorcluster)  [unwired: 16 in]
              }
            }
            n158 = call "Time Delay3"("error in (no error)"=w408) -> ("error out"=w407:errorcluster)  [unwired: 10 in]
            n159 = property on="Load Config" class="Bool (strict)"(error in=w407, "Value"=w412) -> (error out=w409:errorcluster)  [unwired: 1 in, 1 out]
            n160 = property on="Set As Default" class="Bool (strict)"(error in=w409, "Value"=w412) -> (error out=w413:errorcluster)  [unwired: 1 in, 1 out]
          }
          event "Download to Buffer": Value Change {
            n161 = event-data() -> ()  [unwired: 1 in, 5 out]
            n162 = Unbundle By Name(w447) -> ("Operate Status.RF Mode"=w446:u8)
            n163 = case shown="0, Default" w446 {
              selector: w446 -> [w456 w492]
              tunnel: w455 -> [w467 w490]
              tunnel: w454 -> [w466 w491]
              tunnel: [w464 w491] -> w453
              tunnel: [w463 w489] -> w449
              tunnel: [w456 w492] -> _
              frame 0, Default {
                # "0xFFFFFFFFFF to end buffer write"
                # "0 to reset the buffer to starting address\nand enable buffer write"
                n164 = call "sc5511a_list_buffer_write.vi"("deviceHandle"=w466, "List Frequency"=u64 0 ("Frequency"), "error in"=w467) -> ("deviceHandle"=w459:u32, "error out"=w462:errorcluster)  [unwired: 15 in]
                n165 = property on="Frequency List (2048 max)" class="Arr (strict)"(error in=w462) -> (error out=w460:errorcluster, "Value"=w461:u64[])  [unwired: 1 in, 1 out]
                n166 = for {
                  tunnel: w461 -> [w473] mode=indexing
                  tunnel: w460 -> [w475]
                  tunnel: w459 -> [w474]
                  tunnel: [w472] -> w457
                  tunnel: [w471] -> w458
                  i -> [w469]
                  stop <- w470 stop-if-true
                  n167 = Greater?(x=w469, y=2048) -> (0:w470:bool)
                  n168 = case shown="False" w470 {
                    tunnel: w475 -> [w484 w486]
                    tunnel: [w479 w486] -> w471
                    tunnel: w474 -> [w483 w485]
                    tunnel: w473 -> [w482 _]
                    tunnel: [w481 w485] -> w472
                    tunnel: w469 -> [w478 _]
                    frame False {
                      n169 = call "sc5511a_list_buffer_write.vi"("deviceHandle"=w483, "List Frequency"=w482, "error in"=w484) -> ("deviceHandle"=w481:u32, "error out"=w480:errorcluster)  [unwired: 15 in]
                      n170 = Increment(x=w478) -> (x+1=w477:i32)
                      n171 = property on="List Points" class="DigNum (strict)"(error in=w480, "Value"=w477) -> (error out=w479:errorcluster)  [unwired: 1 in, 1 out]
                    }
                    frame True {
                    }
                  }
                }
                n172 = call "sc5511a_list_buffer_write.vi"("deviceHandle"=w457, "List Frequency"=u64 1099511627775 ("Frequency"), "error in"=w458) -> ("deviceHandle"=w464:u32, "error out"=w463:errorcluster)  [unwired: 15 in]
              }
              frame 1 {
                n173 = property on="message 2" class="Str"(error in=w490, "Value"="List/Sweep On" ("message 2"), "Visible"=TRUE) -> (error out=w489:errorcluster)  [unwired: 1 in, 1 out]
              }
            }
            n174 = call "Time Delay2"("error in (no error)"=w449) -> ("error out"=w448:errorcluster)  [unwired: 10 in]
            n175 = property on="Download to Buffer" class="Bool (strict)"(error in=w448, "Value"=FALSE ("Download to Buffer")) -> (error out=w452:errorcluster)  [unwired: 1 in, 1 out]
          }
          event "Save Buffer to EEPROM", "Read EEPROM to Buffer": Value Change {
            w498 = FALSE ("Copy EEPROM to Buffer")
            n176 = event-data() -> ()  [unwired: 1 in, 5 out]
            n177 = Unbundle By Name(w494) -> ("Operate Status.RF Mode"=w493:u8)
            n178 = case shown="0, Default" w493 {
              tunnel: w502 -> [w508 w553]
              tunnel: w501 -> [w507 w555]
              tunnel: [w504 w554] -> w500
              tunnel: [w503 w555] -> w496
              frame 0, Default {
                n179 = property on="Read EEPROM to Buffer" class="Bool (strict)"(error in=w508) -> (error out=w505:errorcluster, "Value"=w506:bool)  [unwired: 1 in, 1 out]
                n180 = case shown="True" w506 {
                  tunnel: w507 -> [w523 w549]
                  tunnel: w505 -> [w517 w548]
                  tunnel: [w519 w547] -> w504
                  tunnel: [w521 w546] -> w503
                  frame True {
                    w524 = u16 1 items=["Buffer to EEPROM", "EEPROM to Buffer"] ("List Eeprom Config")
                    n181 = property on="List Points" class="DigNum (strict)"(error in=w517) -> (error out=w516:errorcluster, "Value"=w515:u32)  [unwired: 1 in, 1 out]
                    n182 = call "sc5511a_list_buffer_transfer.vi"("deviceHandle"=w523, "transfer mode"=w524, "error in"=w516) -> ("deviceHandle"=w520:u32, "error out"=w522:errorcluster)  [unwired: 15 in]
                    n183 = call "Time Delay5"("error in (no error)"=w522) -> ("error out"=w509:errorcluster)  [unwired: 10 in]
                    n184 = Greater Than 0?(x=w515) -> (x > 0?=w514:bool)
                    n185 = case shown="True" w514 {
                      tunnel: w509 -> [w527 w537]
                      tunnel: [w529 w536] -> w521
                      tunnel: w520 -> [w529 w535]
                      tunnel: [w527 w534] -> w518
                      tunnel: [u64[] [] w533] -> w513
                      tunnel: w515 -> [_ w532]
                      tunnel: [0 w531] -> w510
                      tunnel: [0 ("length") 1 ("length")] -> w512
                      frame False {
                      }
                      frame True {
                        n186 = while {
                          tunnel: w537 -> [w545]
                          tunnel: [w544] -> w534
                          tunnel: [w543] -> w536
                          tunnel: w535 -> [w542]
                          tunnel: [w541] -> w533 mode=indexing
                          tunnel: w532 -> [w540]
                          tunnel: [w538] -> w531
                          i -> [w538]
                          stop <- w539 continue-if-true
                          n187 = Less?(x=w538, y=w540) -> (x < y?=w539:bool)
                          n188 = call "sc5511a_list_buffer_read.vi"("deviceHandle"=w542, "address"=w538, "error in"=w545) -> ("deviceHandle"=w543:u32, "frequency"=w541:u64, "error out"=w544:errorcluster)  [unwired: 14 in]
                        }
                      }
                    }
                    n189 = Delete From Array(array=w513, length=w512, index=w510) -> (array with subset deleted=w511:u64[])  [unwired: 1 out]
                    n190 = property on="List Points" class="DigNum (strict)"("Value"=w510) -> ()  [unwired: 2 in, 2 out]
                    n191 = property on="Frequency List (2048 max)" class="Arr (strict)"(error in=w518, "Value"=w511) -> (error out=w519:errorcluster)  [unwired: 1 in, 1 out]
                  }
                  frame False {
                    w550 = u16 0 items=["Buffer to EEPROM", "EEPROM to Buffer"] ("List Eeprom Config")
                    n192 = call "sc5511a_list_buffer_transfer.vi"("deviceHandle"=w549, "transfer mode"=w550, "error in"=w548) -> ("deviceHandle"=w546:u32, "error out"=w547:errorcluster)  [unwired: 15 in]
                  }
                }
              }
              frame 1 {
                n193 = property on="message 2" class="Str"(error in=w553, "Value"="List Mode On" ("message 2"), "Visible"=TRUE) -> (error out=w554:errorcluster)  [unwired: 1 in, 1 out]
              }
            }
            n194 = property on="Read EEPROM to Buffer" class="Bool (strict)"(error in=w500, "Value"=w498) -> (error out=w499:errorcluster)  [unwired: 1 in, 1 out]
            n195 = property on="Save Buffer to EEPROM" class="Bool (strict)"(error in=w499, "Value"=w498) -> (error out=w497:errorcluster)  [unwired: 1 in, 1 out]
          }
        }
        n196 = Greater?(x=w156, y=u32 1500) -> (0:w154:bool)
        n197 = Multiply(x=w152, y=u16 1000) -> (x*y=w150:u16)
        n198 = Greater?(x=w151, y=w150) -> (0:w104:bool)
        n199 = local read "GetStatus"() -> (w148:bool)
        n200 = And(x=w148, y=w104) -> (x .and. y?=w102:bool)
        n201 = Unbundle By Name(w107) -> ("Operate Status.ListRuning"=w106:u8)
        n202 = case shown="True" w102 {
          tunnel: w159 -> [w182 w189]
          tunnel: w158 -> [w181 w188]
          tunnel: [w181 w186] -> w109
          tunnel: [w182 w187] -> w111
          tunnel: [w180 w185] -> w118
          tunnel: w107 -> [w180 _]
          frame False {
          }
          frame True {
            n203 = call "Time Delay6"("error in (no error)"=w188, "Delay Time (s)"=0.005) -> ("error out"=w184:errorcluster)  [unwired: 9 in]
            n204 = call "sc5511a_get_device_status.vi"("deviceHandle"=w189, "error in"=w184) -> ("deviceHandle"=w187:u32, "Device Status"=w185:T11, "error out"=w186:errorcluster)  [unwired: 15 in]
          }
        }
        n205 = Not Equal To 0?(x=w106) -> (x != 0?=w105:bool)
        n206 = And(x=w105, y=w104) -> (x .and. y?=w103:bool)
        n207 = Unbundle By Name(w118) -> ("Operate Status.Lock Mode"=w132:u8, "Operate Status.RFOutState"=w122:u8, "Operate Status.AutoPwrLevel"=w123:u8, "Operate Status.AlcMode"=w124:u8, "Operate Status.RF1 Standby"=w125:u8, "Operate Status.RF Mode"=w126:u8, "Operate Status.ListRuning"=w115:u8, "Operate Status.RF2 Standby"=w127:u8, "Operate Status.Ref Lock Enable"=w128:u8, "Operate Status.ExtRefDetected"=w129:u8, "Operate Status.RefOutSelect"=w130:u8, "PLL Status.Sum PLL"=w131:u8, "PLL Status.Crs assist PLL"=w136:u8, "PLL Status.Crs PLL"=w137:u8, "PLL Status.Crs Ref PLL"=w135:u8, "PLL Status.Fine PLL"=w139:u8, "Operate Status.Device Accessed"=w140:u8, "Operate Status.OverTempStatus"=w141:u8)
        n208 = case shown="True" w103 {
          tunnel: [w164 w171] -> w113
          tunnel: w114 -> [w164 _]
          tunnel: w112 -> [_ w171]
          tunnel: w111 -> [w163 w170]
          tunnel: [w163 w169] -> w110
          tunnel: w109 -> [w162 w168]
          tunnel: [w162 w166] -> w108
          frame False {
          }
          frame True {
            n209 = call "sc5511a_get_temperature.vi"("deviceHandle"=w170, "error in"=w168) -> ("deviceHandle"=w169:u32, "temperature"=w165:sgl, "error out"=w167:errorcluster)  [unwired: 15 in]
            n210 = property on="Temperature" class="DigNum (strict)"(error in=w167, "Value"=w165) -> (error out=w166:errorcluster)  [unwired: 1 in, 1 out]
          }
        }
        n211 = case shown="True" w154 {
          selector: w154 -> [_ w176]
          tunnel: w108 -> [w173 w179]
          tunnel: [w173 w178] -> w143
          tunnel: w146 -> [w172 _]
          tunnel: [w172 w174] -> w147
          tunnel: w112 -> [_ w174]
          frame False {
          }
          frame True {
            n212 = Not(x=w176) -> (.not. x?=w175:bool)
            n213 = property on="message" class="Str"(error in=w179, "Visible"=w175) -> (error out=w177:errorcluster)  [unwired: 1 in, 1 out]
            n214 = property on="message 2" class="Str"(error in=w177, "Visible"=w175) -> (error out=w178:errorcluster)  [unwired: 1 in, 1 out]
          }
        }
        n215 = Not Equal To 0?(x=w132) -> (x != 0?=w133:bool)
        n216 = Select(t=w136, s=w133, f=w137) -> (s? t:f=w134:u8)
        n217 = And(x=w134, y=w135) -> (x .and. y?=w138:u8)
        n218 = Not Equal To 0?(x=w131) -> (x != 0?=w119:bool)
        n219 = Not Equal To 0?(x=w138) -> (x != 0?=w120:bool)
        n220 = Not Equal To 0?(x=w139) -> (x != 0?=w121:bool)
        n221 = Unbundle By Name(w143) -> ("status"=w144:bool)
        n222 = Bundle By Name(cluster=T9 {"Synth Mode"=0, "RF Out"=0, "Auto Power"=0, "ALC Mode"=0, "Standby"=0, "Rf RF Mode"=0, "List Mode State"=0, "RF2 Standby"=0, "Ref Lock Enable"=0, "Ext Ref Detected"=0, "Ref out mode"=0, "Main PLL"=1, "Crs PLL"=1, "Fine PLL"=1, "device accessed"=0, "Over Temp"=0, "MainLED"=FALSE, "CrsLED"=FALSE, "FineLED"=FALSE} ("Device Status"), "Synth Mode"=w132, "RF Out"=w122, "Auto Power"=w123, "ALC Mode"=w124, "Standby"=w125, "Rf RF Mode"=w126, "List Mode State"=w115, "RF2 Standby"=w127, "Ref Lock Enable"=w128, "Ext Ref Detected"=w129, "Ref out mode"=w130, "Main PLL"=w131, "Crs PLL"=w138, "Fine PLL"=w139, "device accessed"=w140, "Over Temp"=w141, "MainLED"=w119, "CrsLED"=w120, "FineLED"=w121) -> (w117:T9)
        n223 = Or(x=w144, y=w145) -> (x .or. y?=w142:bool)
        n224 = property on="Device Status" class="Clust (strict)"("Value"=w117) -> ()  [unwired: 2 in, 2 out]
      }
      n225 = call "sc5511a_close_device.vi"("deviceHandle"=w94, "error in (no error)"=w95) -> ("error out"=w93:errorcluster)  [unwired: 17 in]
      "Selected Resource" <- w79
    }
    frame Error {
    }
  }
  n226 = Unbundle By Name(w6) -> ("status"=w11:bool)
  n227 = case shown="True" w11 {
    selector: w11 -> [_ w557]
    frame False {
    }
    frame True {
      n228 = property on="error out" class="Clust (strict)"("Visible"=w557) -> ()  [unwired: 2 in, 2 out]
      n229 = property on="Tab Control" class="TabCtl (strict)"("Value"=T1."Device Info" ("Tab Control")) -> ()  [unwired: 2 in, 2 out]
    }
  }
  n230 = property on="Selected Resource" class="Str"(error in=w6, "Visible"=w4) -> (error out=w5:errorcluster)  [unwired: 1 in, 1 out]
  n231 = property on="On" class="Bool (strict)"(error in=w5, "Value"=w4) -> (error out=→"error out":errorcluster)  [unwired: 1 in, 1 out]
